vi "auto_jackTime_find.vi"(0 "UL-X":dbl, 1 "x":dbl, 2 "LL-X":dbl, 3 "UL-Y":dbl, 4 "y":dbl, 5 "LL-Y":dbl) -> (17 "?":bool)   [LabVIEW 2019]
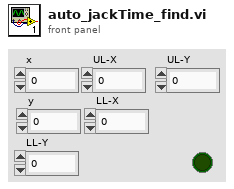
[diagram p1: front panel]
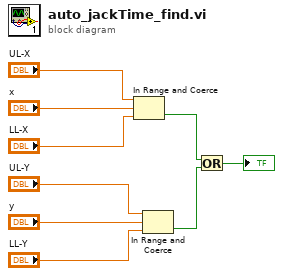
[diagram p0: block diagram]
diagram:
  n1 = In Range and Coerce(upper limit="UL-X", x="x", lower limit="LL-X") -> (In Range?=w3:bool)  [unwired: 1 out]
  n2 = In Range and Coerce(upper limit="UL-Y", x="y", lower limit="LL-Y") -> (In Range?=w2:bool)  [unwired: 1 out]
  n3 = Or(x=w3, y=w2) -> (x .or. y?=→"?":bool)
